vi "-log bis_SD.vi"(1 "Transmission":dbl[](array[numeric])) -> (0 "-log(x)=log(1/x)":dbl[](array[numeric]))   [LabVIEW 2015]
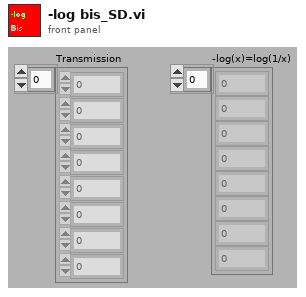
[diagram p1: front panel]
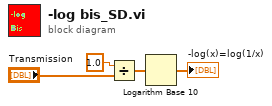
[diagram p0: block diagram]
diagram:
  n1 = Divide(x=1.0, y="Transmission") -> (x/y=w3:dbl[])
  n2 = Logarithm Base 10(1:w3) -> (0:→"-log(x)=log(1/x)":dbl[])
